vi "MOTOR Configure Axis Direction.vi"(8 "error in (no error)":errorcluster, 10 "Message Data":variant, 11 "Data Cluster in":T1={"Tango HW"={"VISA resource"="", "Baud Rate (115200)"=2, "lAnInterfaceType"=0, "bAShowProt"=15}, "Writer Queue"=refnum, "Status"=FALSE, "Abs Position"=[], "Axis Velocity"={"dX"=0.0, "dY"=0.0, "dZ"=0.0, "dA"=0.0}, "acceleration "=0.0, "Z direction"=enum."Up", "Position Mode"="", "plLSID"=0}) -> (0 "error out":errorcluster, 3 "Data Cluster out":T1={"Tango HW"={"VISA resource"="", "Baud Rate (115200)"=2, "lAnInterfaceType"=0, "bAShowProt"=15}, "Writer Queue"=refnum, "Status"=FALSE, "Abs Position"=[], "Axis Velocity"={"dX"=0.0, "dY"=0.0, "dZ"=0.0, "dA"=0.0}, "acceleration "=0.0, "Z direction"=enum."Up", "Position Mode"="", "plLSID"=0})   [LabVIEW 2020, in "MOTOR.lvlib"]
uses:
  MOTOR.lvlib
  PS Hardware Configuration.ctl
  support/Message Queue/Message Cluster.ctl
  support/HW Message Cluster.ctl
  support/PCT FGV CMD.ctl
  support/Message Queue/Message Queue.lvlib
  <instrlib>/Tango_DLL/Tango_DLL.lvlib
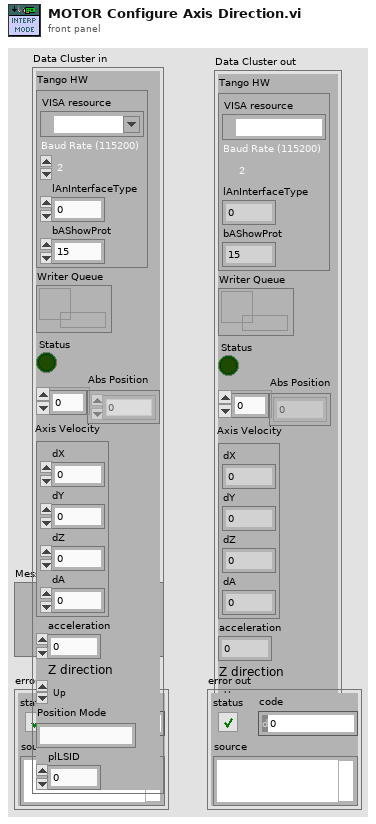
[diagram p1: front panel]
types:
  T1 = typedef "MOTOR.lvlib/PS Hardware Configuration.ctl" = cluster{"Tango HW":cluster{"VISA resource":refnum<visa-resource-name>, "Baud Rate (115200)":i32, "lAnInterfaceType":i32, "bAShowProt":i32}, "Writer Queue":refnum<queue>, "Status":bool, "Abs Position":i32[], "Axis Velocity":cluster{"dX":dbl, "dY":dbl, "dZ":dbl, "dA":dbl}, "acceleration ":dbl, "Z direction":enum16{"Up", "Down"}, "Position Mode":string, "plLSID":i32}
  T2 = typedef "PCT FGV CMD.ctl" = enum16{"INIT", "GET", "SET"}
  T3 = typedef "Message Queue.lvlib/HW Message Cluster.ctl" = cluster{"Writer Queue":refnum<queue>, "Writer Data":T4}
  T4 = typedef "Message Queue.lvlib/Message Cluster.ctl" = cluster{"Message":string, "Message Data":variant}
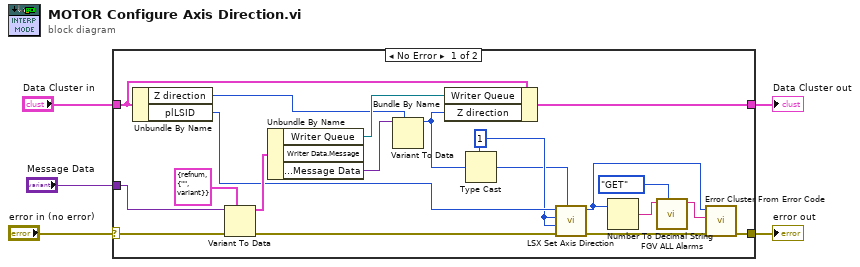
[diagram p0: block diagram]
diagram:
  n1 = case shown="No Error" "error in (no error)" {
    selector: "error in (no error)" -> [w22 w26]
    tunnel: "Message Data" -> [w21 _]
    tunnel: [w20 w27] -> w4
    tunnel: "Data Cluster in" -> [w18 w27]
    tunnel: [w16 w26] -> w2
    frame No Error {
      w10 = 1 ("lZD")
      n2 = Unbundle By Name(w18) -> ("Z direction"=w17:enum16{"Up", "Down"}, "plLSID"=w11:i32)
      n3 = Variant To Data(error in=w22, type=T3 {"Writer Queue"=refnum, "Writer Data"={"Message"="", "Message Data"=variant}}, Variant=w21) -> (data=w25:T3, error out=w7:errorcluster)
      n4 = Unbundle By Name(w25) -> ("Writer Queue"=w24:refnum<queue>, "Writer Data.Message Data"=w19:variant)  [unwired: 1 out]
      n5 = Variant To Data(type=w17, Variant=w19) -> (data=w15:enum16{"Up", "Down"})  [unwired: 1 in, 1 out]
      n6 = Bundle By Name(cluster=w18, "Writer Queue"=w24, "Z direction"=w15) -> (w20:T1)
      n7 = Type Cast(type=w10, x=w15) -> (*(type *) &x=w9:i32)
      n8 = call <instrlib>:"LSX Set Axis Direction.vi"("lZD"=w9, "error in (no error)"=w7, "lYD"=w10, "lXD"=w10, "lLSID"=w11) -> ("error out"=w6:errorcluster, "function return"=w8:i32)  [unwired: 5 in]
      n9 = Number To Decimal String(number=w8) -> (decimal integer string=w13:string)  [unwired: 1 in]
      n10 = call "FGV ALL Alarms.vi"("CMD"=PCT_FGV_CMD."GET", "name"=w13) -> ("Alarm MSG out"=w12:string)  [unwired: 8 in, 1 out]
      n11 = call <vilib>:"Error Cluster From Error Code.vi"("error in (no error)"=w6, "error message (\"\")"=w12, "error code (0)"=w8) -> ("error out"=w16:errorcluster)  [unwired: 6 in]
    }
    frame Error {
    }
  }
  "Data Cluster out" <- w4
  "error out" <- w2
